vi "encodeUInt.vi"(8 "error in (no error)":errorcluster, 10 "Variant":variant) -> (0 "error out":errorcluster, 2 "Array":u8[](array[numeric]) format="%.0x")   [LabVIEW 2016, in "MsgPack.lvlib"]
uses:
  MsgPack.lvlib
  <vilib>/Utility/Data Type/NI_Data Type.lvlib
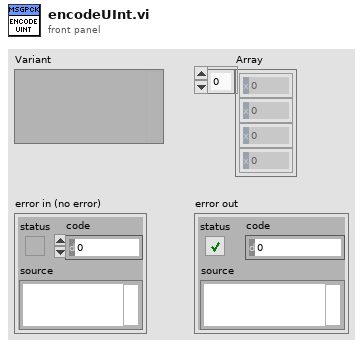
[diagram p1: front panel]
types:
  T1 = typedef "NI_Data Type.lvlib/Data Type.ctl" = enum8{"Invalid Type", "Void", "I8", "I16", "I32", "I64", "U8", "U16", "U32", "U64", "Single Float", "Double Float", "Extended Float", "Single Complex", "Double Complex", "Extended Complex", "Enum U8", "Enum U16", "Enum U32", "Enum U64", "Single Float With Unit", "Double Float With Unit", "Extended Float With Unit", "Single Complex with Unit", "Double Complex with Unit", "Extended Complex with Unit", "Boolean", "String", "Path", "Picture", "Tag", "Array", "Cluster", "Variant", "LV Variant", "Waveform", "Timestamp", "Digital Waveform", "Digital Data", "ExpressData", "Refnum", "External Data", "VI", "Poly VI", "LabVIEW Class Instance", "Fixed Point"}
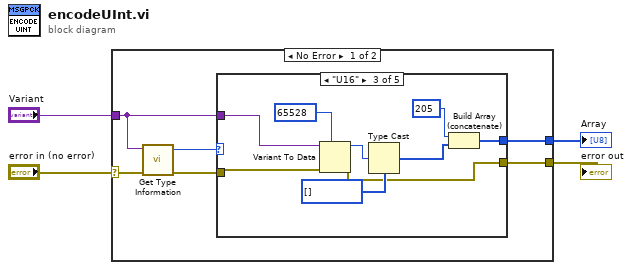
[diagram p0: block diagram]
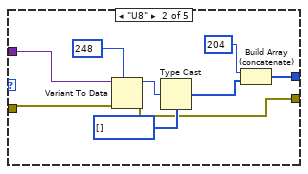
[diagram p3: hidden frame]
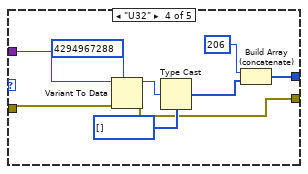
[diagram p4: hidden frame]
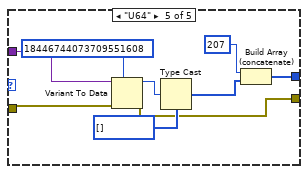
[diagram p5: hidden frame]
diagram:
  n1 = case shown="No Error" "error in (no error)" {
    selector: "error in (no error)" -> [w5 w48]
    tunnel: "Variant" -> [w8 _]
    tunnel: [w7 _] -> w3
    tunnel: [w6 w48] -> w2
    frame No Error {
      n2 = call <vilib>:"Get Type Information.vi"("error in (no error)"=w5, "Variant"=w8) -> ("error out"=w9:errorcluster, "Type"=w10:T1)  [unwired: 5 in, 3 out]
      n3 = case shown="\"U16\"" w10 {
        tunnel: w9 -> [w11 w20 w29 w38 w47]
        tunnel: w8 -> [_ w19 w28 w37 w46]
        tunnel: [_ w13 w22 w31 w40] -> w7
        tunnel: [w11 w12 w21 w30 w39] -> w6
        frame "Invalid Type", Default {
        }
        frame "U8" {
          n4 = Variant To Data(error in=w20, type=u8 248, Variant=w19) -> (data=w16:u8, error out=w12:errorcluster)
          n5 = Type Cast(type=u8[] [], x=w16) -> (*(type *) &x=w14:u8[])
          n6 = Build Array (concatenate)(u8 204, w14) -> (w13:u8[])
        }
        frame "U16" {
          n7 = Variant To Data(error in=w29, type=u16 65528, Variant=w28) -> (data=w25:u16, error out=w21:errorcluster)
          n8 = Type Cast(type=u8[] [], x=w25) -> (*(type *) &x=w23:u8[])
          n9 = Build Array (concatenate)(u8 205, w23) -> (w22:u8[])
        }
        frame "U32" {
          n10 = Variant To Data(error in=w38, type=u32 4294967288, Variant=w37) -> (data=w34:u32, error out=w30:errorcluster)
          n11 = Type Cast(type=u8[] [], x=w34) -> (*(type *) &x=w32:u8[])
          n12 = Build Array (concatenate)(u8 206, w32) -> (w31:u8[])
        }
        frame "U64" {
          n13 = Variant To Data(error in=w47, type=u64 18446744073709551608, Variant=w46) -> (data=w43:u64, error out=w39:errorcluster)
          n14 = Type Cast(type=u8[] [], x=w43) -> (*(type *) &x=w41:u8[])
          n15 = Build Array (concatenate)(u8 207, w41) -> (w40:u8[])
        }
      }
    }
    frame Error {
    }
  }
  "Array" <- w3
  "error out" <- w2
